vi "Mission Controller Send State.vi"(8 "error in (no error)":errorcluster, 11 "RDS Mission Controller Actor in":refnum<class "RDS Mission Controller Actor.lvclass">) -> (0 "error out":errorcluster, 3 "RDS Mission Controller Actor out":refnum<class "RDS Mission Controller Actor.lvclass">)   [LabVIEW 2015, in "RDS Mission Controller Actor.lvlib" / "RDS Mission Controller Actor.lvclass"]
uses:
  RDS Mission Controller Actor.lvclass
  Libraries/RDS Child Messages/Mission Messages/Mission Controller State Message.lvclass
  Libraries/RDS Framework/RDS Message ID.ctl
  Libraries/RDS Child Messages/Mission Messages/Mission Controller State Control.ctl
  Mission Controller Navigation State.ctl
  MissionOp.ctl
  RDS Mission Controller Actor.lvclass/RDS Mission Controller Actor.ctl
  Libraries/RDS Framework/RDS Message Class/RDS Message.lvclass/RDS Message.ctl
  Libraries/RDS Child Messages/Mission Messages/Mission Controller State Message.lvclass/Mission Controller State Message.ctl
  Libraries/RDS Framework/RDS Message Class/RDS Message.lvclass
  Libraries/RDS Child Messages/RDS Child Messages.lvlib
  RDS Mission Controller Actor.lvlib
  Actors/RDS Parent Actor/RDS Parent Actor/RDS Parent Actor.lvclass
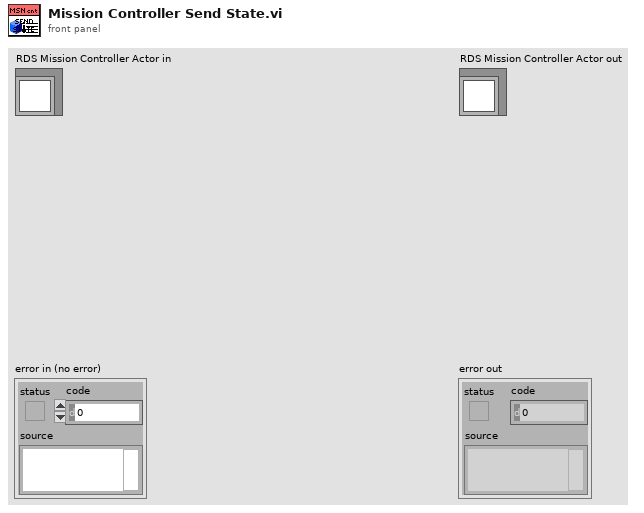
[diagram p1: front panel]
types:
  T1 = typedef "RDS Child Messages.lvlib/Mission Controller State Message.lvclass/Mission Controller State Control.ctl" = cluster{"iHasControl":bool, "controlTimer":timestamp, "Nav State":T2, "Current MissionOp Index":i32, "Mission":T3[], "Distance to Target":dbl, "Seconds to Timeout":dbl}
  T2 = typedef "RDS Mission Controller Actor.lvlib/Mission Controller Navigation State.ctl" = cluster{"GPS Latitude":ext, "GPS Longitude":ext, "Compass Heading":dbl, "Speed":dbl}
  T3 = typedef "RDS Mission Controller Actor.lvlib/MissionOp.ctl" = cluster{"MissionOp Type":enum16{"Waypoint", "Loiter", "Wait", "Deploy AIP", "Stow AIP"}, "Duration (s)":u16, "Throttle":i16, "GPS Latitude":dbl, "GPS Longitude":dbl, "Loiter Range (m)":u16}
  T4 = typedef "RDS Child Messages.lvlib/RDS Message ID.ctl" = enum16{"RDS Hello World", "String Message", "AIP_Status", "AIP_Command", "GPS_Data", "MCB_Command", "MCB_Status", "Compass_Data", "Depth_Data", "Battery_Data", "Contoller_State", "Set_Mag_Dev", "BTB_Shutdown", "State_Sample_Request", "State_Sample", "PID_Gains_Set", "Helm_Limiter_Set", "Helm_Heading_Command", "Helm_Steering_Command", "Helm_Status", "Controller_Message", "AIP_Set_Min_Depth", "Mission_Controller_State", "Mission_Upload", "Mission_Set_Op_and_Run", "Mission_Settings_Set"}
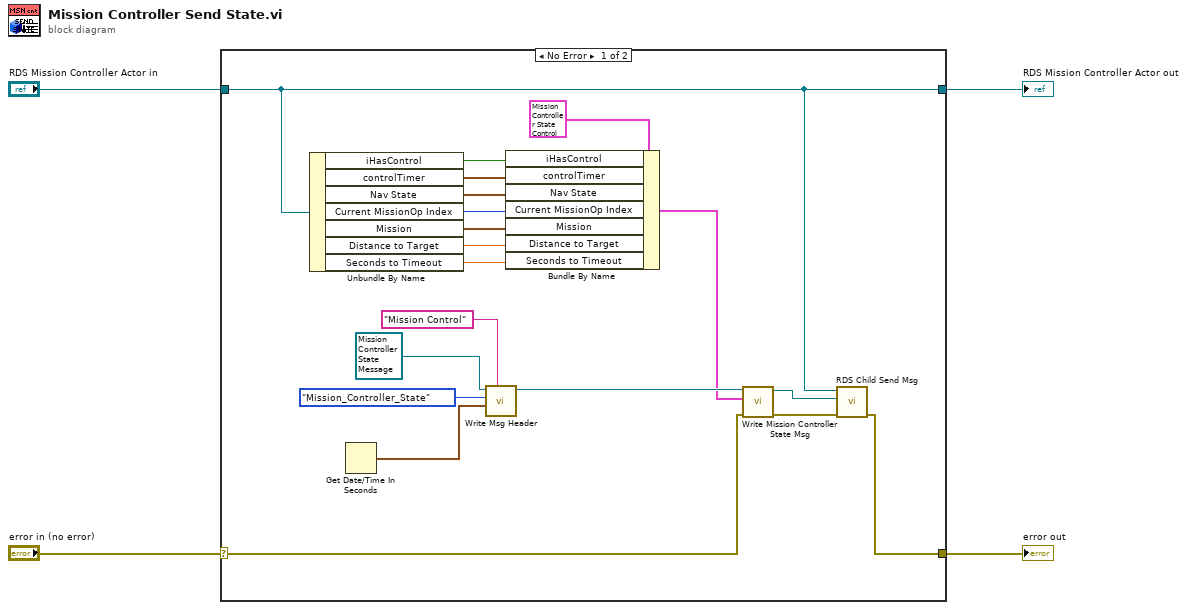
[diagram p0: block diagram]
diagram:
  n1 = case shown="No Error" "error in (no error)" {
    selector: "error in (no error)" -> [w6 w25]
    tunnel: [w5 w25] -> w3
    tunnel: [w9 w24] -> w1
    tunnel: "RDS Mission Controller Actor in" -> [w9 w24]
    frame No Error {
      n2 = Unbundle By Name(w9) -> ("iHasControl"=w16:bool, "controlTimer"=w15:timestamp, "Nav State"=w14:T2, "Current MissionOp Index"=w13:i32, "Mission"=w12:T3[], "Distance to Target"=w8:dbl, "Seconds to Timeout"=w7:dbl)
      n3 = Get Date/Time In Seconds() -> (seconds since 1Jan1904=w23:timestamp)
      n4 = call "Write Msg Header.vi"("Sender Name"="Mission Control", "Time Stamp"=w23, "Msg ID"=RDS_Message_ID."Mission_Controller_State", "RDS Message in"=refnum<class "Mission Controller State Message.lvclass"> refnum ("RDS Child Messages.lvlib:Mission Controller State Message.lvclass")) -> ("RDS Message out"=w19:refnum<class "Mission Controller State Message.lvclass">)  [unwired: 6 in, 1 out]
      n5 = Bundle By Name(cluster=T1 {"iHasControl"=FALSE, "controlTimer"=timestamp(0 s since 1904-01-01), "Nav State"={"GPS Latitude"=0.0, "GPS Longitude"=0.0, "Compass Heading"=0.0, "Speed"=0.0}, "Current MissionOp Index"=0, "Mission"=[], "Distance to Target"=0.0, "Seconds to Timeout"=0.0} ("Mission Controller State"), "iHasControl"=w16, "controlTimer"=w15, "Nav State"=w14, "Current MissionOp Index"=w13, "Mission"=w12, "Distance to Target"=w8, "Seconds to Timeout"=w7) -> (w17:T1)
      n6 = call "Write Mission Controller State Msg.vi"("error in (no error)"=w6, "Mission Controller State"=w17, "Mission Controller State Message in"=w19) -> ("error out"=w11:errorcluster, "Mission Controller State Message out"=w10:refnum<class "Mission Controller State Message.lvclass">)  [unwired: 7 in]
      n7 = call "RDS Child Send Msg.vi"("error in (no error)"=w11, "RDS Message"=w10, "RDS Parent Actor in"=w9) -> ("error out"=w5:errorcluster)  [unwired: 7 in, 1 out]
    }
    frame Error {
    }
  }
  "error out" <- w3
  "RDS Mission Controller Actor out" <- w1
